vi "Start Time Data.vi"(8 "error in (no error)":errorcluster, 9 "Start Time":timestamp, 11 "Function":string) -> (0 "Error Out":errorcluster, 1 "Start Time":timestamp, 3 "Start Time (String)":string)   [LabVIEW 2015, in "Exposure Process.lvlib"]
uses:
  Exposure Process.lvlib
  <vilib>/addons/PointValueMap/PointValueMap.lvlib
  <vilib>/addons/PointValueMap/subVIs/Point_Read_variant.vi
  <vilib>/addons/PointValueMap/subVIs/Point_Write_variant.vi
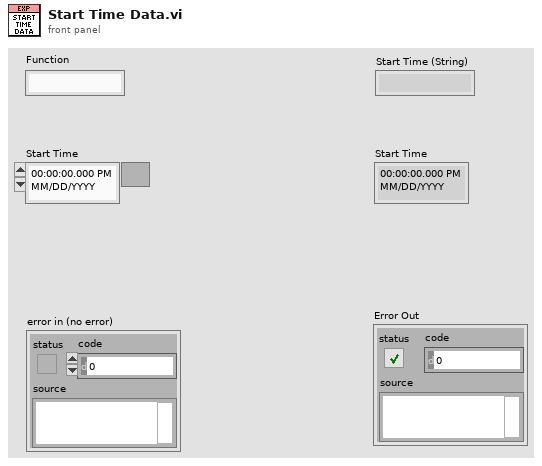
[diagram p1: front panel]
types:
  T1 = typedef "PointValueMap.lvlib/PointMap.ctl" = refnum<data-value>
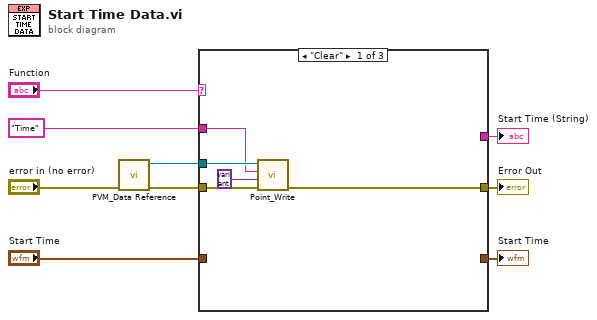
[diagram p0: block diagram]
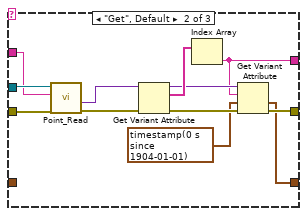
[diagram p2: hidden frame]
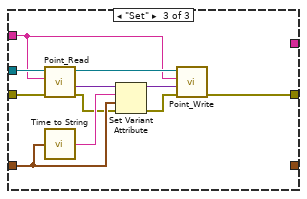
[diagram p3: hidden frame]
diagram:
  n1 = call "PVM_Data Reference.vi"("error in (no error)"="error in (no error)") -> ("error out"=w7:errorcluster, "Map Out"=w8:T1)  [unwired: 9 in]
  n2 = case shown="\"Clear\"" "Function" {
    tunnel: w8 -> [w14 w26 w37]
    tunnel: w7 -> [w13 w25 w36]
    tunnel: "Start Time" -> [_ _ w33]
    tunnel: "Time" -> [w11 w24 w30]
    tunnel: [w12 w19 w27] -> w1
    tunnel: [_ w16 _] -> w3
    tunnel: [_ w15 _] -> w2
    frame "Clear" {
      n3 = call-poly <vilib>:"Point_Write.vi"("Error In"=w13, "Value"=variant, "Tag"=w11, "Map"=w14) -> ("Error Out"=w12:errorcluster)  [unwired: 6 in, 1 out]
    }
    frame "Get", Default {
      n4 = call-poly <vilib>:"Point_Read.vi"("Error In"=w25, "Tag"=w24, "Map"=w26) -> ("Error Out"=w23:errorcluster, "Value"=w22:variant)  [unwired: 3 in, 4 out]
      n5 = Get Variant Attribute(Variant=w22, error in=w23) -> (duplicate Variant=w20:variant, names=w21:string[], error out=w18:errorcluster)  [unwired: 2 in, 1 out]
      n6 = Index Array(array=w21) -> (element=w16:string)  [unwired: 1 in]
      n7 = Get Variant Attribute(Variant=w20, name=w16, default value (empty Variant)=timestamp(0 s since 1904-01-01), error in=w18) -> (value=w15:timestamp, error out=w19:errorcluster)  [unwired: 2 out]
    }
    frame "Set" {
      n8 = call-poly <vilib>:"Point_Read.vi"("Error In"=w36, "Tag"=w30, "Map"=w37) -> ("Error Out"=w29:errorcluster, "Value"=w35:variant, "Map Out"=w32:T1)  [unwired: 3 in, 3 out]
      n9 = call "Time to String.vi"("Time Stamp"=w33) -> ("date/time string"=w34:string)
      n10 = Set Variant Attribute(Variant=w35, name=w34, value=w33, error in=w29) -> (Variant out=w31:variant, error out=w28:errorcluster)  [unwired: 1 out]
      n11 = call-poly <vilib>:"Point_Write.vi"("Error In"=w28, "Value"=w31, "Tag"=w30, "Map"=w32) -> ("Error Out"=w27:errorcluster)  [unwired: 6 in, 1 out]
    }
  }
  "Start Time (String)" <- w3
  "Start Time" <- w2
  "Error Out" <- w1
